vi "Data Ref FGV.vi"(7 "Command":T2, 8 "error in (no error)":errorcluster, 9 "Output Length":i32, 10 "Input Length":i32, 11 "Device Ref in":T1 format="%.0x") -> (0 "error out":errorcluster, 1 "Output FIFO Index / Length":i32, 2 "Input FIFO Index / Length":i32, 3 "Device Ref out":T1 format="%.0x")   [LabVIEW 2019, in "SEECD Engine.lvlib"]
uses:
  SEECD Engine.lvlib
  <vilib>/NI VeriStand/Custom Device API/Custom Device Item Ref.ctl
  Type Defs/Data Ref FGV Command.ctl
  <vilib>/NI VeriStand/Custom Device API/Custom Device API.lvlib
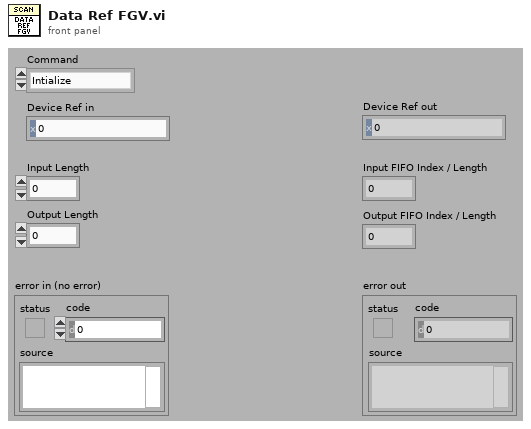
[diagram p1: front panel]
types:
  T1 = typedef "Custom Device API.lvlib/Custom Device Item Ref.ctl" = u64
  T2 = typedef "SEECD Engine.lvlib/Data Ref FGV Command.ctl" = enum16{"Intialize", "Get", "Update"}
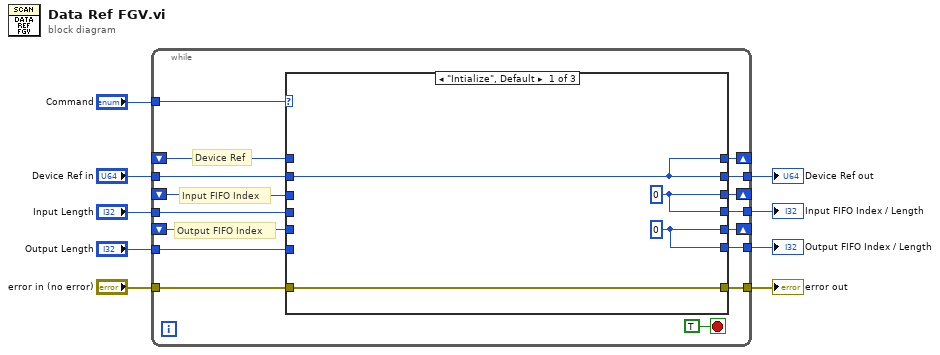
[diagram p0: block diagram]
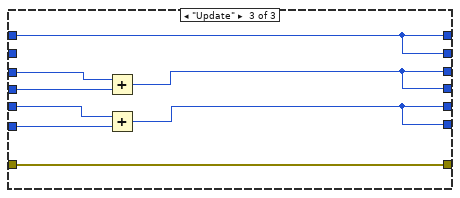
[diagram p3: hidden frame]
diagram:
  n1 = while {
    shift-right: [w23] -> _
    shift-left: _ -> [w20]
    tunnel: "Command" -> [w25]
    tunnel: "Device Ref in" -> [w24]
    shift-right: [w21] -> _
    shift-left: _ -> [w19]
    shift-right: [w17] -> _
    shift-left: _ -> [w18]
    tunnel: "Input Length" -> [w16]
    tunnel: "Output Length" -> [w15]
    tunnel: [w14] -> w5
    tunnel: [w13] -> w4
    tunnel: [w12] -> w3
    tunnel: "error in (no error)" -> [w11]
    tunnel: [w10] -> w1
    stop <- TRUE stop-if-true
    # "Output FIFO Index"
    # "Input FIFO Index"
    # "Device Ref"
    n2 = case shown="\"Intialize\", Default" w25 {
      tunnel: w24 -> [w27 _ _]
      tunnel: [w27 w32 w37] -> w23
      tunnel: [w29 w31 w36] -> w21
      tunnel: w20 -> [_ w32 w37]
      tunnel: w19 -> [_ w31 w40]
      tunnel: w18 -> [_ w33 w38]
      tunnel: [w28 w33 w35] -> w17
      tunnel: w16 -> [_ _ w41]
      tunnel: w15 -> [_ _ w39]
      tunnel: [w27 w32 w37] -> w14
      tunnel: [w29 w31 w36] -> w13
      tunnel: [w28 w33 w35] -> w12
      tunnel: w11 -> [w26 w30 w34]
      tunnel: [w26 w30 w34] -> w10
      frame "Intialize", Default {
        w28 = 0 ("index")
        w29 = 0 ("index")
      }
      frame "Get" {
      }
      frame "Update" {
        n3 = Add(x=w40, y=w41) -> (x+y=w36:i32)
        n4 = Add(x=w38, y=w39) -> (x+y=w35:i32)
      }
    }
  }
  "Device Ref out" <- w5
  "Input FIFO Index / Length" <- w4
  "Output FIFO Index / Length" <- w3
  "error out" <- w1
